vi "rule editor.vi"() -> (0 "output descriptions out":string[][](array[string]), 1 "State names":string[](array[string]), 3 "rule file":path, 4 "output descriptions out 2":string[][](array[string]))   [LabVIEW 2012]
uses:
  rule.ctl
  condition.ctl
  greater or less.ctl
  toolbar icons/Save configuration.ctl
  toolbar icons/open configuration.ctl
  toolbar icons/help.ctl
  variable setpoint.ctl
  data ave interval.ctl
  type specifier for control code.ctl
  rules.ctl
  State rules.ctl
  Output control.ctl
  logic buffer cmd.ctl
  DAC project/Calibration and Function folders.ctl
  calibration/global scale array.vi
panel:
  in  "Tab Control":enum32{"Set Points", "Rules & States"}(tab)
  in  "Configure Function":bool
  in  "Calculate set point":bool
  out "Required Sensors":i32(listbox)
  out "Required Set Points":i32(listbox)
  out "code match":bool
  out "data match":bool
  in  "S P & V definitions":T1[](array[typedef]) {"value" format="%#_6p"; "variable"."Data average interval" min=0.0 format="%^#_3g"}
  in  "add set point before":bool
  in  "delete set point":bool
  in  "add set point after":bool
  in  "Set Points and Variables List":i32(listbox)=1
  in  "Tab states and rules":enum32{"Rules", "States"}(tab)
  in  "Rules":T4=[{"state rules"=[{"next state"=0, "conditions"=[], "number of conditions"=0, "Rule name"=""}, {"next state"=1, "conditions"=[{"> or <"=FALSE, "set point"=500, "sensors and variables"=0, "Data average interval"=0.0}], "number of conditions"=1, "Rule name"=""}, {"next state"=1, "conditions"=[{"> or <"=FALSE, "set point"=10, "sensors and variables"=0, "Data average interval"=0.0}, {"> or <"=FALSE, "set point"=10, "sensors and variables"=0, "Data average interval"=0.0}, {"> or <"=TRUE, "set point"=20, "sensors and variables"=0, "Data average interval"=0.0}, {"> or <"=TRUE, "set point"=500, "sensors and variables"=0, "Data average interval"=0.0}], "number of conditions"=4, "Rule name"=""}], "State name"=""}, {"state rules"=[{"next state"=1, "conditions"=[{"> or <"=FALSE, "set point"=0, "sensors and variables"=0, "Data average interval"=0.0}], "number of conditions"=1, "Rule name"=""}, {"next state"=0, "conditions"=[{"> or <"=FALSE, "set point"=0, "sensors and variables"=0, "Data average interval"=0.0}], "number of conditions"=4, "Rule name"=""}], "State name"=""}] {"state rules"."number of conditions" min=1 step=1; "state rules"."conditions"."Data average interval" min=0.0 format="%^#_3g"; "state rules"."conditions"."sensors and variables" items=["Elapsed time in current state", ""]; "state rules"."conditions"."set point" items=["OFF", "ON"]; "state rules"."next state" items=["OFF"]}
  in  "output descriptions":string[][](array[string])
  in  "output settings":T9 items=["OFF", "ON"]
  in  "add rule before":bool
  in  "delete rule":bool
  in  "add rule after":bool
  in  "Rule List":i32(listbox)
  in  "add state before":bool
  in  "delete state":bool
  in  "add state after":bool
  in  "State List":i32(listbox)
  in  "Help Button":T10
  out "Sensor names":string[](array[string])
  in  "Open logic":T11
  in  "Save logic":T12
  in  "new rule":cluster{"state rules":T6[], "State name":string}={"state rules"=[{"next state"=0, "conditions"=[{"> or <"=FALSE, "set point"=0, "sensors and variables"=0, "Data average interval"=0.0}], "number of conditions"=1, "Rule name"="New Rule"}], "State name"="New State"} {"state rules"."number of conditions" min=1 step=1; "state rules"."conditions"."Data average interval" min=0.0 format="%^#_3g"; "state rules"."conditions"."sensors and variables" items=["Elapsed time in current state"]; "state rules"."next state" items=["john", "dick"]}
  in  "OK Button":bool
  out "Unit":string[](array[string])
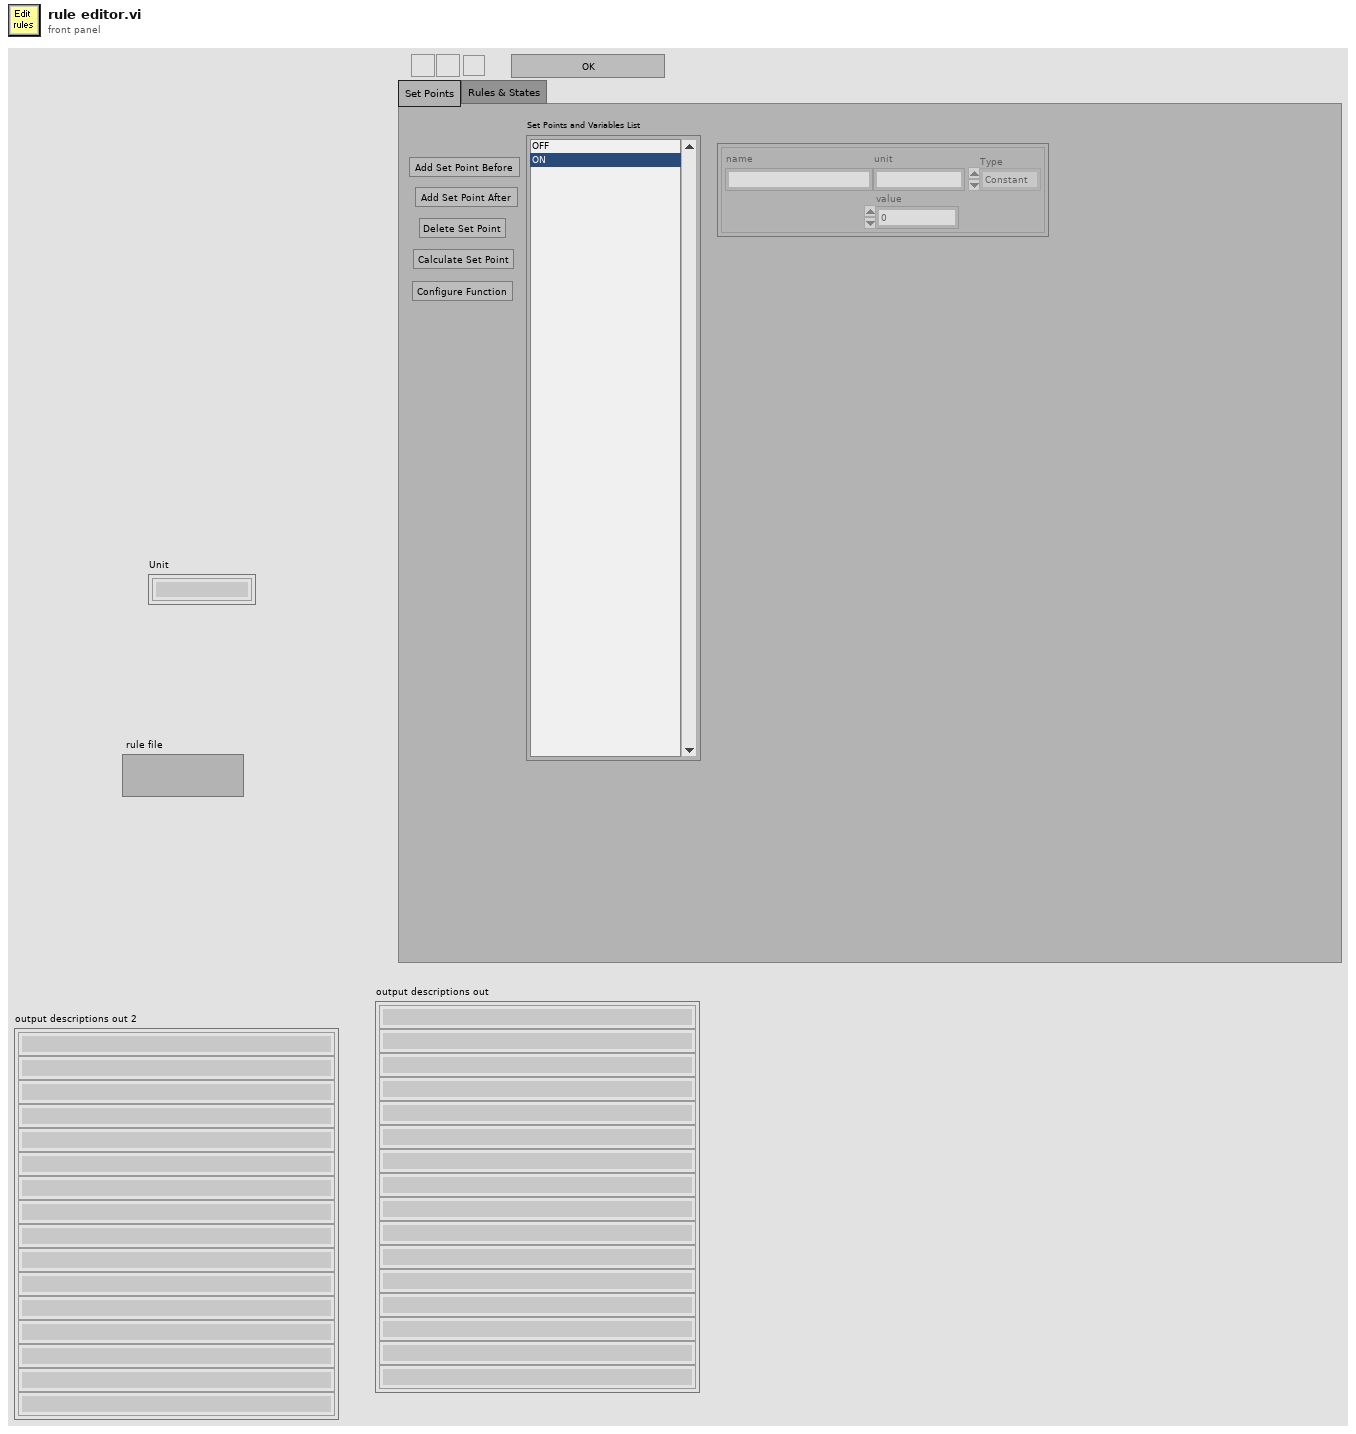
[diagram p1: front panel]
types:
  T1 = typedef "variable setpoint.ctl" = cluster{"name":string, "unit":string, "value":dbl, "Type":enum16{"Constant", "Variable"}, "variable":cluster{"selected sensors":i32[], "selected set points":i32[], "VI":path, "Data average interval":T2, "code ref":T3}}
  T2 = typedef "data ave interval.ctl" = dbl
  T3 = typedef "type specifier for control code.ctl" = refnum<vi>
  T4 = typedef "rules.ctl" = T5[]
  T5 = typedef "State rules.ctl" = cluster{"state rules":T6[], "State name":string}
  T6 = typedef "rule.ctl" = cluster{"next state":u16, "conditions":T7[], "number of conditions":u8, "Rule name":string}
  T7 = typedef "condition.ctl" = cluster{"> or <":T8, "set point":i32, "sensors and variables":i32, "Data average interval":dbl}
  T8 = typedef "greater or less.ctl" = bool
  T9 = typedef "Output control.ctl" = u16[][]
  T10 = typedef "help.ctl" = bool
  T11 = typedef "open configuration.ctl" = bool
  T12 = typedef "Save configuration.ctl" = bool
  T13 = typedef "Calibration and Function folders.ctl" = enum16{"Sensors", "Functions", "Config File", "UserAppFolder"}
  T14 = typedef "logic buffer cmd.ctl" = enum16{"read", "write ouput settings", "write rules", "write setpoints", "write output descriptions", "write all", "calculate setpoints", "save", "open", "Load all setpoint code", "Load one setpoint code", "Configure one setpoint code"}
  T15 = typedef "setpoint match.ctl" = cluster{"required data":cluster{"Set Point names":string[], "required number of setpoints":u8, "required number of sensors":u8, "Sensor names":string[]}, "input match":bool, "code match":bool, "variable?":bool}
  T16 = typedef "calib array.ctl" = T17[]
  T17 = typedef "conversion.ctl" = cluster{"conversion matrix":sgl[][], "units":string, "name":string, "scale type":T18, "offset (volts)":dbl, "second channel":i8, "correspondence table":T19, "offset (physical units)":dbl, "pH scale":T20, "D.O.":T21}
  T18 = typedef "scale type.ctl" = enum16{"Volts", "Polynomial", "Correspondence Table", "pH", "Dissolved Oxygen", "Quadratic"}
  T19 = typedef "correspondence table.ctl" = cluster{"physical units":dbl, "volts":dbl}[]
  T20 = typedef "pH scale.ctl" = cluster{"Buffers":cluster{"Buffer":dbl, "Calibrated":bool, "V/T":dbl}[], "Temperature":dbl}
  T21 = typedef "DO scale.ctl" = cluster{"Temperature":dbl, "K":dbl, "barometric pressure":dbl}
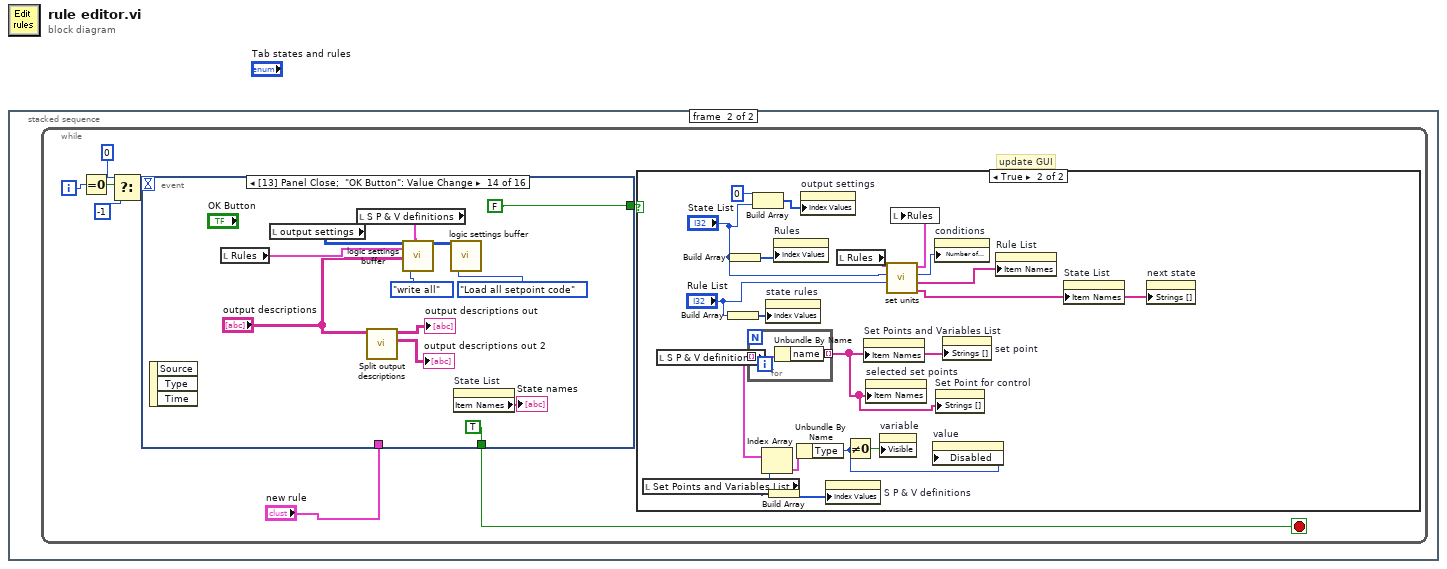
[diagram p0: block diagram]
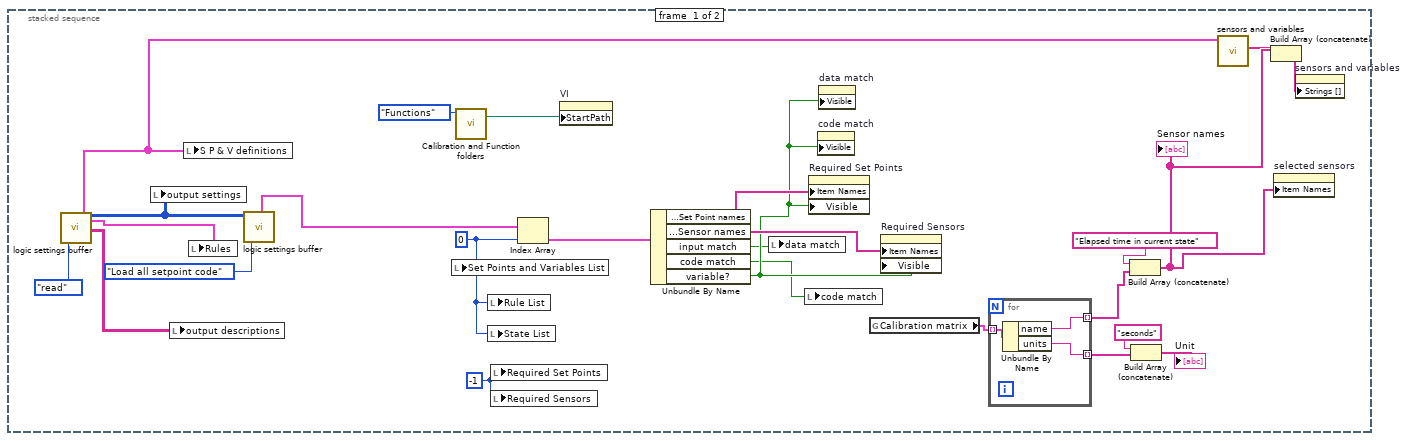
[diagram p2: hidden frame]
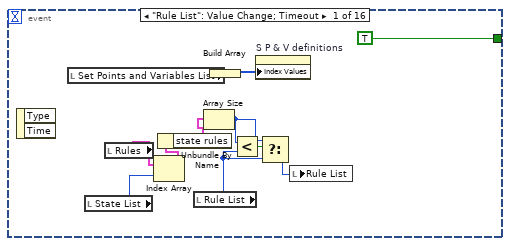
[diagram p4: hidden frame]
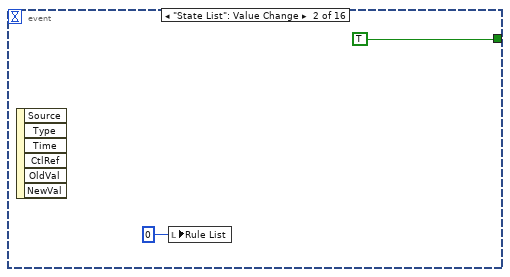
[diagram p5: hidden frame]
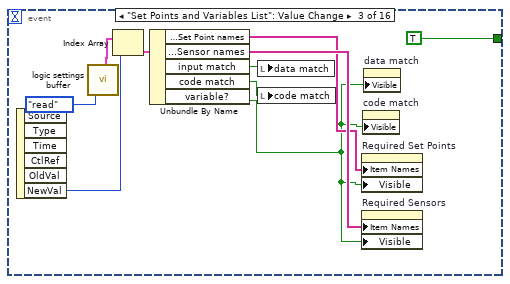
[diagram p6: hidden frame]
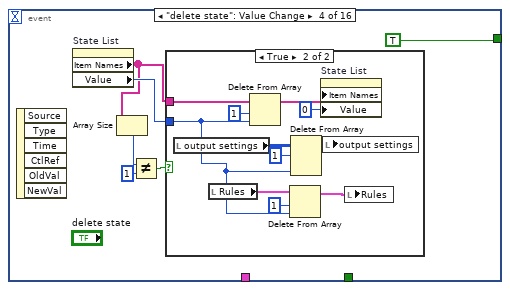
[diagram p7: hidden frame]
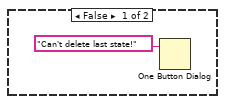
[diagram p8: hidden frame]
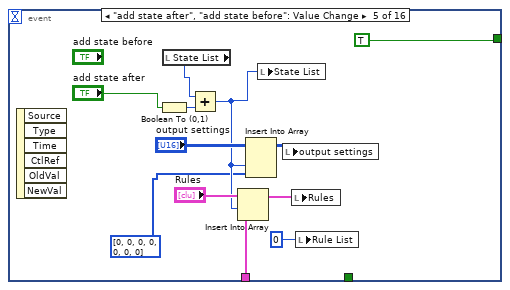
[diagram p9: hidden frame]
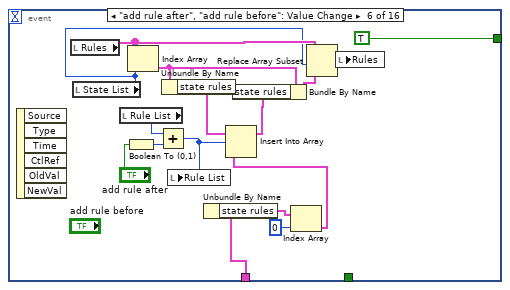
[diagram p10: hidden frame]
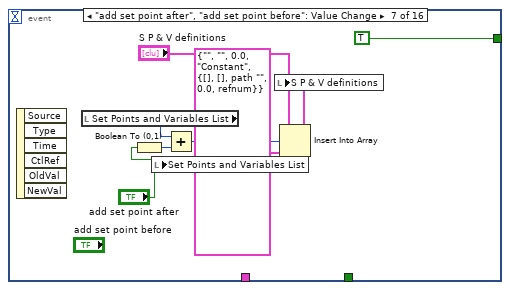
[diagram p11: hidden frame]
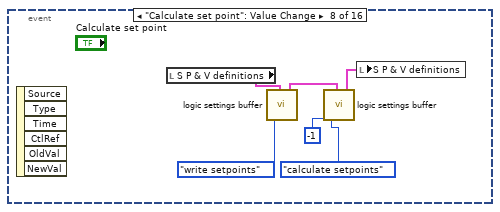
[diagram p12: hidden frame]
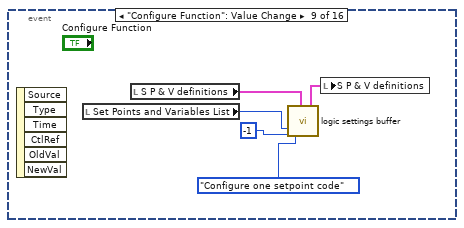
[diagram p13: hidden frame]
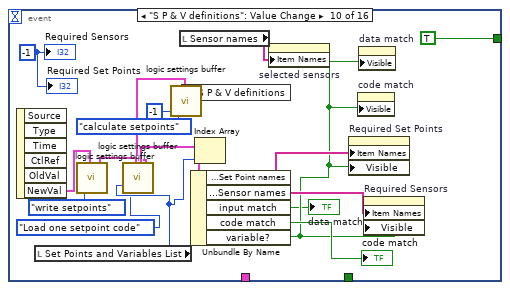
[diagram p14: hidden frame]
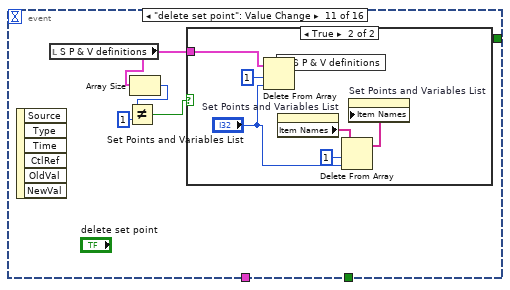
[diagram p15: hidden frame]
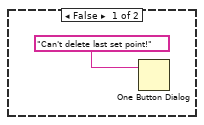
[diagram p16: hidden frame]
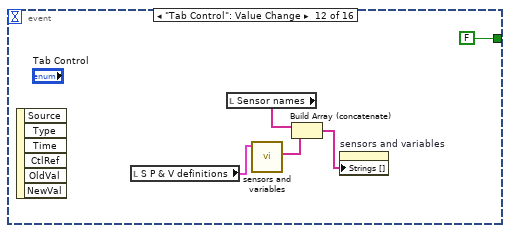
[diagram p17: hidden frame]
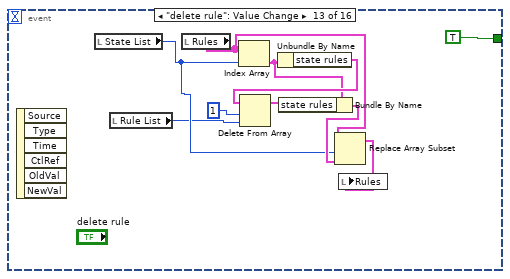
[diagram p18: hidden frame]
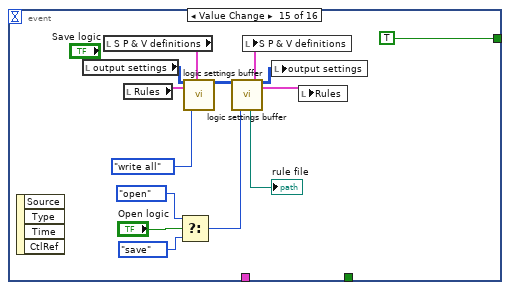
[diagram p19: hidden frame]
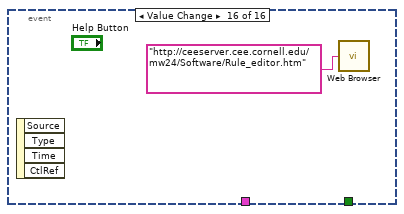
[diagram p20: hidden frame]
diagram:
  n1 = stacked-sequence {
    frame #0 {
      w12 = -1 ("Required Sensors")
      w11 = 0 ("Current Set Point")
      n2 = call "logic settings buffer.vi"("command"=logic_buffer_cmd."read") -> ("Set Points out"=w6:T1[], "ouput settings out"=w19:T9, "Rules out"=w22:T4, "output descriptions out"=w21:string[][])  [unwired: 11 in, 4 out]
      n3 = local write "output settings"(w19) -> ()
      n4 = local write "output descriptions"(w21) -> ()
      n5 = local write "S P & V definitions"(w6) -> ()
      n6 = local write "Rules"(w22) -> ()
      n7 = call "logic settings buffer.vi"("output settings"=w19, "command"=logic_buffer_cmd."Load all setpoint code") -> ("Setpoint match"=w7:T15[])  [unwired: 10 in, 7 out]
      n8 = local write "Set Points and Variables List"(w11) -> ()
      n9 = call "Calibration and Function folders.vi"("Folder"=Calibration_and_Function_folders."Functions") -> ("Selected Folder"=w1:path)  [unwired: 10 in]
      n10 = local write "Rule List"(w11) -> ()
      n11 = local write "State List"(w11) -> ()
      n12 = local write "Required Set Points"(w12) -> ()
      n13 = local write "Required Sensors"(w12) -> ()
      n14 = Index Array(array=w7, index=w11) -> (element=w16:T15)
      n15 = property on="VI" class="Path"("StartPath"=w1) -> ()  [unwired: 2 in, 2 out]
      n16 = Unbundle By Name(w16) -> ("required data.Set Point names"=w18:string[], "required data.Sensor names"=w17:string[], "input match"=w13:bool, "code match"=w14:bool, "variable?"=w15:bool)
      n17 = local write "data match"(w13) -> ()
      n18 = local write "code match"(w14) -> ()
      n19 = property on="Required Set Points" class="LstBox (strict)"("Item Names"=w18, "Visible"=w15) -> ()  [unwired: 2 in, 2 out]
      n20 = property on="code match" class="Bool (strict)"("Visible"=w15) -> ()  [unwired: 2 in, 2 out]
      n21 = property on="data match" class="Bool (strict)"("Visible"=w15) -> ()  [unwired: 2 in, 2 out]
      n22 = global read "global scale array.vi" "Calibration matrix"() -> (w26:T16)
      n23 = property on="Required Sensors" class="LstBox (strict)"("Item Names"=w17, "Visible"=w15) -> ()  [unwired: 2 in, 2 out]
      n24 = for {
        tunnel: w26 -> [w29] mode=indexing
        tunnel: [w28] -> w25 mode=indexing
        tunnel: [w27] -> w10 mode=indexing
        n25 = Unbundle By Name(w29) -> ("name"=w27:string, "units"=w28:string)
      }
      n26 = Build Array (concatenate)("Elapsed time in current state" ("name"), w10) -> (w4:string[])
      "Sensor names" <- w4
      n27 = Build Array (concatenate)("seconds" ("name"), w25) -> (→"Unit":string[])
      n28 = call "sensors and variables.vi"("S P & V definitions"=w6) -> ("Variable names"=w3:string[])  [unwired: 7 in, 3 out]
      n29 = Build Array (concatenate)(w4, w3) -> (w5:string[])
      n30 = property on="selected sensors" class="LstBox (strict)"("Item Names"=w4) -> ()  [unwired: 2 in, 2 out]
      n31 = property on="sensors and variables" class="Ring (strict)"("Strings []"=w5) -> ()  [unwired: 2 in, 2 out]
    }
    frame #1 {
      n32 = while {
        i -> [w36]
        stop <- w37 stop-if-true
        # "update GUI"
        n33 = Equal To 0?(x=w36) -> (x = 0?=w35:bool)
        n34 = Select(t=0, s=w35, f=-1) -> (s? t:f=w30:i32)
        n35 = event shown="[13] Panel Close;  \"OK Button\": Value Change" {
          selector: _ -> [_ _ _ _ _ _ _ _ _ _ _ _ _ _ _ _]
          dyn-events: _ -> [_ _ _ _ _ _ _ _ _ _ _ _ _ _ _ _]
          timeout: w30 -> [_ _ _ _ _ _ _ _ _ _ _ _ _ _ _ _]
          tunnel: [_ _ _ _ _ _ _ _ _ _ _ _ _ TRUE _ _] -> w37
          tunnel: [TRUE TRUE TRUE TRUE TRUE TRUE TRUE _ _ TRUE _ FALSE TRUE FALSE TRUE _] -> w32
          tunnel: "new rule" -> [_ _ _ _ w104 w117 _ _ _ _ _ _ _ _ _ _]
          event "Rule List": Value Change; Timeout {
            n36 = event-data() -> ()  [unwired: 1 in, 2 out]
            n37 = local read "Set Points and Variables List"() -> (w59:i32)
            n38 = local read "State List"() -> (w63:i32)
            n39 = local read "Rules"() -> (w60:T4)
            n40 = Index Array(array=w60, index=w63) -> (element=w62:T5)
            n41 = Unbundle By Name(w62) -> ("state rules"=w61:T6[])
            n42 = local read "Rule List"() -> (w64:i32)
            n43 = Array Size(array=w61) -> (size(s)=w65:i32)
            n44 = Build Array(w59) -> (w58:i32[])
            n45 = Less?(x=w65, y=w64) -> (x < y?=w67:bool)
            n46 = property on="S P & V definitions" class="Arr (strict)"("Index Values"=w58) -> ()  [unwired: 2 in, 2 out]
            n47 = Select(t=w65, s=w67, f=w64) -> (s? t:f=w66:i32)
            n48 = local write "Rule List"(w66) -> ()
          }
          event "State List": Value Change {
            n49 = event-data() -> ()  [unwired: 1 in, 6 out]
            n50 = local write "Rule List"(0 ("Current Rule")) -> ()
          }
          event "Set Points and Variables List": Value Change {
            n51 = event-data() -> ("NewVal"=w71:i32)  [unwired: 1 in, 5 out]
            n52 = call "logic settings buffer.vi"("command"=logic_buffer_cmd."read") -> ("Setpoint match"=w72:T15[])  [unwired: 11 in, 7 out]
            n53 = Index Array(array=w72, index=w71) -> (element=w74:T15)
            n54 = Unbundle By Name(w74) -> ("required data.Set Point names"=w78:string[], "required data.Sensor names"=w79:string[], "input match"=w75:bool, "code match"=w76:bool, "variable?"=w77:bool)
            n55 = local write "data match"(w75) -> ()
            n56 = local write "code match"(w76) -> ()
            n57 = property on="Required Set Points" class="LstBox (strict)"("Item Names"=w78, "Visible"=w77) -> ()  [unwired: 2 in, 2 out]
            n58 = property on="Required Sensors" class="LstBox (strict)"("Item Names"=w79, "Visible"=w77) -> ()  [unwired: 2 in, 2 out]
            n59 = property on="code match" class="Bool (strict)"("Visible"=w77) -> ()  [unwired: 2 in, 2 out]
            n60 = property on="data match" class="Bool (strict)"("Visible"=w77) -> ()  [unwired: 2 in, 2 out]
          }
          event "delete state": Value Change {
            n61 = event-data() -> ()  [unwired: 1 in, 6 out]
            n62 = property on="State List" class="LstBox (strict)"() -> ("Item Names"=w84:string[], "Value"=w85:i32)  [unwired: 2 in, 2 out]
            n63 = Array Size(array=w84) -> (size(s)=w82:i32)
            n64 = Not Equal?(x=w82, y=1) -> (x != y?=w83:bool)
            n65 = case shown="True" w83 {
              tunnel: w84 -> [_ w94]
              tunnel: w85 -> [_ w88]
              frame False {
                n66 = One Button Dialog(message="Can't delete last state!") -> ()  [unwired: 1 in, 1 out]
              }
              frame True {
                n67 = local read "output settings"() -> (w97:T9)
                n68 = local read "Rules"() -> (w92:T4)
                n69 = Delete From Array(array=w94, length=1, index=w88) -> (array with subset deleted=w90:string[])  [unwired: 1 out]
                n70 = Delete From Array(array=w92, length=1, index=w88) -> (array with subset deleted=w91:T4)  [unwired: 1 out]
                n71 = Delete From Array(array=w97, length=1, index (col)=w88) -> (array with subset deleted=w98:T9)  [unwired: 1 in, 1 out]
                n72 = property on="State List" class="LstBox (strict)"("Item Names"=w90, "Value"=0 ("Current State")) -> ()  [unwired: 2 in, 2 out]
                n73 = local write "output settings"(w98) -> ()
                n74 = local write "Rules"(w91) -> ()
              }
            }
          }
          event "add state after", "add state before": Value Change {
            n75 = event-data() -> ()  [unwired: 1 in, 6 out]
            n76 = Boolean To (0,1)(Boolean="add state after") -> (0, 1=w109:i16)
            n77 = local read "State List"() -> (w103:i32)
            n78 = Add(x=w103, y=w109) -> (x+y=w100:i32)
            n79 = Insert Into Array(array="Rules", index=w100, new element=w104) -> (w107:T4)
            n80 = Insert Into Array(array="output settings", index (col)=w100, new element=u16[] [0, 0, 0, 0, 0, 0, 0] ("new element/subarray")) -> (w110:T9)  [unwired: 1 in]
            n81 = local write "State List"(w100) -> ()
            n82 = local write "output settings"(w110) -> ()
            n83 = local write "Rules"(w107) -> ()
            n84 = local write "Rule List"(0 ("Current Rule")) -> ()
          }
          event "add rule after", "add rule before": Value Change {
            n85 = event-data() -> ()  [unwired: 1 in, 6 out]
            n86 = local read "Rules"() -> (w113:T4)
            n87 = local read "State List"() -> (w112:i32)
            n88 = local read "Rule List"() -> (w123:i32)
            n89 = Boolean To (0,1)(Boolean="add rule after") -> (0, 1=w124:i16)
            n90 = Index Array(array=w113, index=w112) -> (element=w121:T5)
            n91 = Add(x=w123, y=w124) -> (x+y=w111:i32)
            n92 = Unbundle By Name(w121) -> ("state rules"=w120:T6[])
            n93 = local write "Rule List"(w111) -> ()
            n94 = Unbundle By Name(w117) -> ("state rules"=w116:T6[])
            n95 = Index Array(array=w116, index=0) -> (element=w115:T6)
            n96 = Insert Into Array(array=w120, index=w111, new element=w115) -> (w119:T6[])
            n97 = Bundle By Name(cluster=w121, "state rules"=w119) -> (w118:T5)
            n98 = Replace Array Subset(array=w113, new element=w118, index=w112) -> (w122:T4)
            n99 = local write "Rules"(w122) -> ()
          }
          event "add set point after", "add set point before": Value Change {
            n100 = event-data() -> ()  [unwired: 1 in, 6 out]
            n101 = local read "Set Points and Variables List"() -> (w133:i32)
            n102 = Boolean To (0,1)(Boolean="add set point after") -> (0, 1=w134:i16)
            n103 = Add(x=w133, y=w134) -> (x+y=w129:i32)
            n104 = local write "Set Points and Variables List"(w129) -> ()
            n105 = Insert Into Array(array="S P & V definitions", index=w129, new element=T1 {"name"="", "unit"="", "value"=0.0, "Type"=enum."Constant", "variable"={"selected sensors"=[], "selected set points"=[], "VI"=path "", "Data average interval"=0.0, "code ref"=refnum}} ("new element/subarray")) -> (w131:T1[])
            n106 = local write "S P & V definitions"(w131) -> ()
          }
          event "Calculate set point": Value Change {
            n107 = event-data() -> ()  [unwired: 1 in, 6 out]
            n108 = local read "S P & V definitions"() -> (w139:T1[])
            n109 = call "logic settings buffer.vi"("command"=logic_buffer_cmd."write setpoints", "Set Points"=w139) -> ("Set Points out"=w138:T1[])  [unwired: 10 in, 7 out]
            n110 = call "logic settings buffer.vi"("Plant  state"=-1, "command"=logic_buffer_cmd."calculate setpoints", "Set Points"=w138) -> ("Set Points out"=w137:T1[])  [unwired: 9 in, 7 out]
            n111 = local write "S P & V definitions"(w137) -> ()
          }
          event "Configure Function": Value Change {
            n112 = event-data() -> ()  [unwired: 1 in, 6 out]
            n113 = local read "Set Points and Variables List"() -> (w141:i32)
            n114 = local read "S P & V definitions"() -> (w143:T1[])
            n115 = call "logic settings buffer.vi"("index"=w141, "Plant  state"=-1, "command"=logic_buffer_cmd."Configure one setpoint code", "Set Points"=w143) -> ("Set Points out"=w145:T1[])  [unwired: 8 in, 7 out]
            n116 = local write "S P & V definitions"(w145) -> ()
          }
          event "S P & V definitions": Value Change {
            w160 = -1 ("Required Sensors")
            n117 = event-data() -> ("NewVal"=w151:T1[])  [unwired: 1 in, 5 out]
            n118 = local read "Set Points and Variables List"() -> (w157:i32)
            n119 = call "logic settings buffer.vi"("command"=logic_buffer_cmd."write setpoints", "Set Points"=w151) -> ("Set Points out"=w158:T1[])  [unwired: 10 in, 7 out]
            n120 = call "logic settings buffer.vi"("index"=w157, "command"=logic_buffer_cmd."Load one setpoint code", "Set Points"=w158) -> ("Setpoint match"=w156:T15[], "Set Points out"=w149:T1[])  [unwired: 9 in, 6 out]
            n121 = call "logic settings buffer.vi"("Plant  state"=-1, "command"=logic_buffer_cmd."calculate setpoints", "Set Points"=w149) -> ("Set Points out"=w148:T1[])  [unwired: 9 in, 7 out]
            n122 = local read "Sensor names"() -> (w163:string[])
            n123 = local write "S P & V definitions"(w148) -> ()
            n124 = Index Array(array=w156, index=w157) -> (element=w155:T15)
            n125 = Unbundle By Name(w155) -> ("required data.Set Point names"=w162:string[], "required data.Sensor names"=w161:string[], "input match"=→"data match":bool, "code match"=→"code match":bool, "variable?"=w153:bool)
            n126 = property on="selected sensors" class="LstBox (strict)"("Item Names"=w163) -> ()  [unwired: 2 in, 2 out]
            n127 = property on="Required Set Points" class="LstBox (strict)"("Item Names"=w162, "Visible"=w153) -> ()  [unwired: 2 in, 2 out]
            n128 = property on="code match" class="Bool (strict)"("Visible"=w153) -> ()  [unwired: 2 in, 2 out]
            n129 = property on="data match" class="Bool (strict)"("Visible"=w153) -> ()  [unwired: 2 in, 2 out]
            n130 = property on="Required Sensors" class="LstBox (strict)"("Item Names"=w161, "Visible"=w153) -> ()  [unwired: 2 in, 2 out]
            "Required Set Points" <- w160
            "Required Sensors" <- w160
          }
          event "delete set point": Value Change {
            n131 = event-data() -> ()  [unwired: 1 in, 6 out]
            n132 = local read "S P & V definitions"() -> (w167:T1[])
            n133 = Array Size(array=w167) -> (size(s)=w166:i32)
            n134 = Not Equal?(x=w166, y=1) -> (x != y?=w165:bool)
            n135 = case shown="True" w165 {
              tunnel: w167 -> [_ w174]
              frame False {
                n136 = One Button Dialog(message="Can't delete last set point!") -> ()  [unwired: 1 in, 1 out]
              }
              frame True {
                n137 = Delete From Array(array=w174, length=1, index="Set Points and Variables List") -> (array with subset deleted=w175:T1[])  [unwired: 1 out]
                n138 = local write "S P & V definitions"(w175) -> ()
                n139 = property on="Set Points and Variables List" class="LstBox (strict)"() -> ("Item Names"=w173:string[])  [unwired: 2 in, 2 out]
                n140 = Delete From Array(array=w173, length=1, index="Set Points and Variables List") -> (array with subset deleted=w172:string[])  [unwired: 1 out]
                n141 = property on="Set Points and Variables List" class="LstBox (strict)"("Item Names"=w172) -> ()  [unwired: 2 in, 2 out]
              }
            }
          }
          event "Tab Control": Value Change {
            n142 = event-data() -> ()  [unwired: 1 in, 6 out]
            n143 = local read "S P & V definitions"() -> (w180:T1[])
            n144 = local read "Sensor names"() -> (w178:string[])
            n145 = call "sensors and variables.vi"("S P & V definitions"=w180) -> ("Variable names"=w179:string[])  [unwired: 7 in, 3 out]
            n146 = Build Array (concatenate)(w178, w179) -> (w177:string[])
            n147 = property on="sensors and variables" class="Ring (strict)"("Strings []"=w177) -> ()  [unwired: 2 in, 2 out]
          }
          event "delete rule": Value Change {
            n148 = event-data() -> ()  [unwired: 1 in, 6 out]
            n149 = local read "State List"() -> (w183:i32)
            n150 = local read "Rule List"() -> (w182:i32)
            n151 = local read "Rules"() -> (w187:T4)
            n152 = Index Array(array=w187, index=w183) -> (element=w189:T5)
            n153 = Unbundle By Name(w189) -> ("state rules"=w190:T6[])
            n154 = Delete From Array(array=w190, length=1, index=w182) -> (array with subset deleted=w188:T6[])  [unwired: 1 out]
            n155 = Bundle By Name(cluster=w189, "state rules"=w188) -> (w185:T5)
            n156 = Replace Array Subset(array=w187, new element=w185, index=w183) -> (w186:T4)
            n157 = local write "Rules"(w186) -> ()
          }
          event Panel Close; "OK Button": Value Change {
            n158 = event-data() -> ()  [unwired: 1 in, 3 out]
            n159 = local read "Rules"() -> (w199:T4)
            n160 = local read "output settings"() -> (w200:T9)
            n161 = local read "S P & V definitions"() -> (w198:T1[])
            n162 = call "Split output descriptions.vi"("output descriptions combined"="output descriptions") -> ("output descriptions 2"=→"output descriptions out 2":string[][], "output descriptions"=→"output descriptions out":string[][])  [unwired: 9 in]
            n163 = call "logic settings buffer.vi"("output settings"=w200, "Rules"=w199, "output descriptions"="output descriptions", "command"=logic_buffer_cmd."write all", "Set Points"=w198) -> ("ouput settings out"=w195:T9)  [unwired: 7 in, 7 out]
            n164 = call "logic settings buffer.vi"("output settings"=w195, "command"=logic_buffer_cmd."Load all setpoint code") -> ()  [unwired: 10 in, 8 out]
            n165 = property on="State List" class="LstBox (strict)"() -> ("Item Names"=→"State names":string[])  [unwired: 2 in, 2 out]
          }
          event Value Change {
            n166 = event-data() -> ()  [unwired: 1 in, 4 out]
            n167 = local read "output settings"() -> (w206:T9)
            n168 = local read "S P & V definitions"() -> (w207:T1[])
            n169 = local read "Rules"() -> (w205:T4)
            n170 = Select(t=logic_buffer_cmd."open" ("command"), s="Open logic", f=logic_buffer_cmd."save" ("command")) -> (s? t:f=w214:T14)
            n171 = call "logic settings buffer.vi"("output settings"=w206, "Rules"=w205, "command"=logic_buffer_cmd."write all", "Set Points"=w207) -> ("ouput settings out"=w209:T9)  [unwired: 8 in, 7 out]
            n172 = call "logic settings buffer.vi"("output settings"=w209, "command"=w214) -> ("Set Points out"=w212:T1[], "rule file out"=→"rule file":path, "ouput settings out"=w213:T9, "Rules out"=w211:T4)  [unwired: 10 in, 4 out]
            n173 = local write "S P & V definitions"(w212) -> ()
            n174 = local write "output settings"(w213) -> ()
            n175 = local write "Rules"(w211) -> ()
          }
          event Value Change {
            n176 = event-data() -> ()  [unwired: 1 in, 4 out]
            n177 = call "Web Browser.vi"("URL"="http://ceeserver.cee.cornell.edu/mw24/Software/Rule_editor.htm") -> ()  [unwired: 1 in]
          }
        }
        n178 = case shown="True" w32 {
          frame False {
          }
          frame True {
            n179 = local read "Set Points and Variables List"() -> (w47:i32)
            n180 = local read "S P & V definitions"() -> (w48:T1[])
            n181 = Build Array("Rule List") -> (w55:i32[])
            n182 = Build Array("State List") -> (w45:i32[])
            n183 = for {
              tunnel: w48 -> [w57] mode=indexing
              tunnel: [w56] -> w41 mode=indexing
              n184 = Unbundle By Name(w57) -> ("name"=w56:string)
            }
            n185 = Build Array(0 ("element"), "State List") -> (w43:i32[])
            n186 = Index Array(array=w48, index=w47) -> (element=w46:T1)
            n187 = property on="state rules" class="Arr (strict)"("Index Values"=w55) -> ()  [unwired: 2 in, 2 out]
            n188 = Build Array(w47) -> (w49:i32[])
            n189 = property on="Rules" class="Arr (strict)"("Index Values"=w45) -> ()  [unwired: 2 in, 2 out]
            n190 = Unbundle By Name(w46) -> ("Type"=w39:enum16{"Constant", "Variable"})
            n191 = property on="output settings" class="Arr (strict)"("Index Values"=w43) -> ()  [unwired: 2 in, 2 out]
            n192 = property on="S P & V definitions" class="Arr (strict)"("Index Values"=w49) -> ()  [unwired: 2 in, 2 out]
            n193 = local read "Rules"() -> (w50:T4)
            n194 = Not Equal To 0?(x=w39) -> (x != 0?=w40:bool)
            n195 = property on="Set Points and Variables List" class="LstBox (strict)"("Item Names"=w41) -> ()  [unwired: 2 in, 2 out]
            n196 = property on="selected set points" class="LstBox (strict)"("Item Names"=w41) -> ()  [unwired: 2 in, 2 out]
            n197 = property on="variable" class="Clust (strict)"("Visible"=w40) -> ()  [unwired: 2 in, 2 out]
            n198 = call "set units.vi"("Current Rule"="Rule List", "Current State"="State List", "Rules"=w50) -> ("State names"=w51:string[], "Rule names"=w52:string[], "number of conditions"=w38:u8, "Rules out"=w54:T4)  [unwired: 1 in]
            n199 = local write "Rules"(w54) -> ()
            n200 = property on="value" class="DigNum (strict)"("Disabled"=w39) -> ()  [unwired: 2 in, 2 out]
            n201 = property on="conditions" class="Arr (strict)"("Number of Rows"=w38) -> ()  [unwired: 2 in, 2 out]
            n202 = property on="Set Point for control" class="Ring (strict)"("Strings []"=w41) -> ()  [unwired: 2 in, 2 out]
            n203 = property on="set point" class="Ring (strict)"("Strings []"=w41) -> ()  [unwired: 2 in, 2 out]
            n204 = property on="Rule List" class="LstBox (strict)"("Item Names"=w52) -> ()  [unwired: 2 in, 2 out]
            n205 = property on="State List" class="LstBox (strict)"("Item Names"=w51) -> ()  [unwired: 2 in, 2 out]
            n206 = property on="next state" class="Ring (strict)"("Strings []"=w51) -> ()  [unwired: 2 in, 2 out]
          }
        }
      }
    }
  }
